vi "UpdateVariableGroups.vi"(8 "error in (no error)":errorcluster, 11 "VMUI in":refnum<class "VMUI.lvclass">) -> (0 "error out":errorcluster, 3 "VMUI out":refnum<class "VMUI.lvclass">)   [LabVIEW 2013, in "VMUI.lvclass"]
uses:
  VMUI.lvclass
  VariableManager/VariableManager.lvclass
  VariableGroup/VariableGroup.lvclass
  API/VariableManagerAPI.lvlib
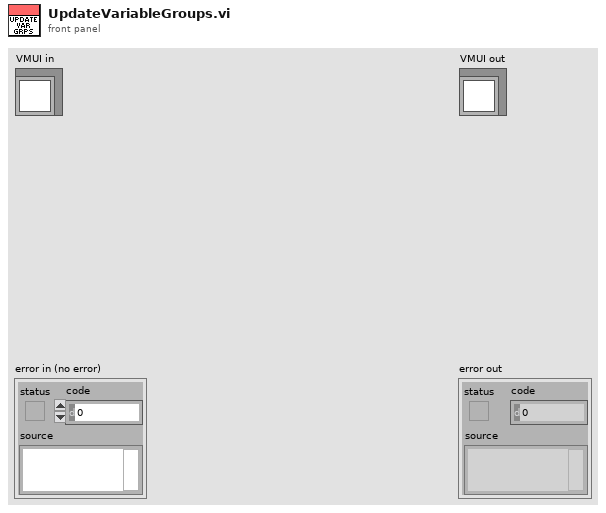
[diagram p1: front panel]
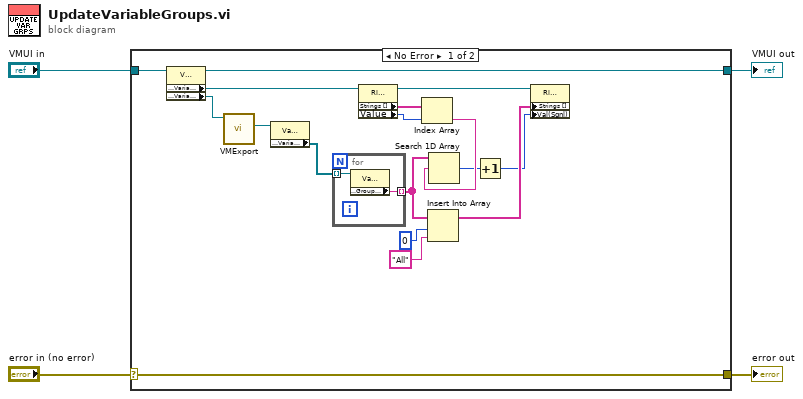
[diagram p0: block diagram]
diagram:
  n1 = case shown="No Error" "error in (no error)" {
    selector: "error in (no error)" -> [w21 w25]
    tunnel: [w21 w25] -> w3
    tunnel: [w9 w24] -> w1
    tunnel: "VMUI in" -> [w20 w24]
    frame No Error {
      n2 = property class="VMUI.lvclass"(reference=w20) -> (reference out=w9:refnum<class "VMUI.lvclass">, "Accessors:VariableGroupRingRef"=w13:refnum<vi>, "Accessors:VariableManagerRef"=w7:refnum<vi>)  [unwired: 1 in, 1 out]
      n3 = call "VMExport.vi"("VariableManagerRef in"=w7) -> ("VariableManagerExportCopy"=w6:refnum<class "VariableManager.lvclass">)  [unwired: 8 in, 2 out]
      n4 = property class="VariableManager.lvclass"(reference=w6) -> ("Accessors:VariableGroups"=w8:refnum<class "VariableGroup.lvclass">[])  [unwired: 1 in, 2 out]
      n5 = for {
        tunnel: w8 -> [w23] mode=indexing
        tunnel: [w22] -> w17 mode=indexing
        n6 = property class="VariableGroup.lvclass"(reference=w23) -> ("Accessors:GroupName"=w22:string)  [unwired: 1 in, 2 out]
      }
      n7 = property class="Ring (strict)"(reference=w13) -> (reference out=w5:refnum<vi>, "Strings []"=w19:string[], "Value"=w10:u16)  [unwired: 1 in, 1 out]
      n8 = Index Array(array=w19, index=w10) -> (element=w18:string)
      n9 = Insert Into Array(array=w17, index=0, new element="All") -> (w12:string[])
      n10 = Search 1D Array(1D array=w17, element=w18) -> (index of element=w14:i32)  [unwired: 1 in]
      n11 = Increment(x=w14) -> (x+1=w11:i32)
      n12 = property class="Ring (strict)"(reference=w5, "Strings []"=w12, "Val(Sgnl)"=w11) -> ()  [unwired: 1 in, 2 out]
    }
    frame Error {
    }
  }
  "error out" <- w3
  "VMUI out" <- w1
